vi "GoDeepSleep.vi"(6 "Resp Timeout (ms)":i32 min=0, 7 "Enum":T1, 8 "Error In":errorcluster, 11 "FPGA Reference":refnum<k20>) -> (0 "Error Out":errorcluster, 1 "Received Text":string, 2 "Deep Sleep OK":bool)   [LabVIEW 2018]
uses:
  Resources_Test/UART/ControlTestSlot.ctl
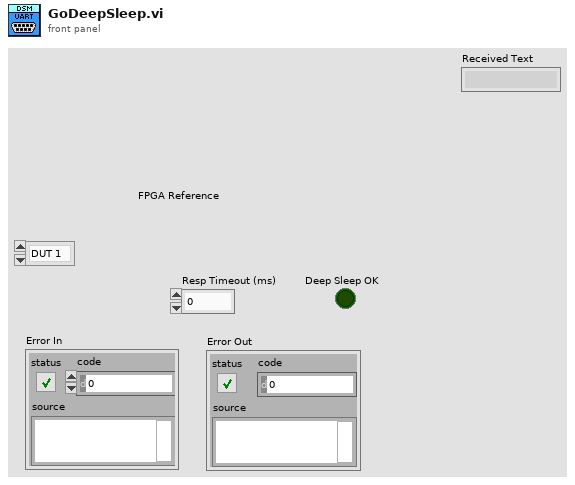
[diagram p1: front panel]
types:
  T1 = typedef "ControlTestSlot.ctl" = enum16{"DUT 1", "DUT 2"}
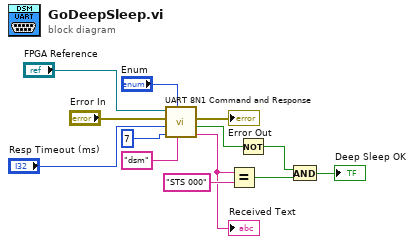
[diagram p0: block diagram]
diagram:
  n1 = call "UART 8N1 Command and Response.vi"("Text to Send"="dsm", "Active Dut"="Enum", "Response Size (char)"=u32 7, "Response Timeout (ms)"="Resp Timeout (ms)", "Error In"="Error In", "FPGA VI Reference In"="FPGA Reference") -> ("Received Text"=w7:string, "Timeout Flag"=w5:bool, "Error Out"=→"Error Out":errorcluster)  [unwired: 1 in, 2 out]
  "Received Text" <- w7
  n2 = Equal?(x=w7, y="STS 000") -> (x = y?=w6:bool)
  n3 = Not(x=w5) -> (.not. x?=w4:bool)
  n4 = And(x=w4, y=w6) -> (x .and. y?=→"Deep Sleep OK":bool)
